vi "Raise WebMessage Received Event.vi"(4 "Event in":refnum<user-event>, 5 "Event Data":cluster{"sender":refnum<k24>, "e":refnum<k24>}, 6 "Control Ref":refnum<k24>, 7 "Event Common Data":T1) -> ()   [LabVIEW 2020, in "WebView.lvclass"]
uses:
  WebView.lvclass
  <vilib>/sklein/WebView2/Libs/Microsoft.Web.WebView2.Core.dll
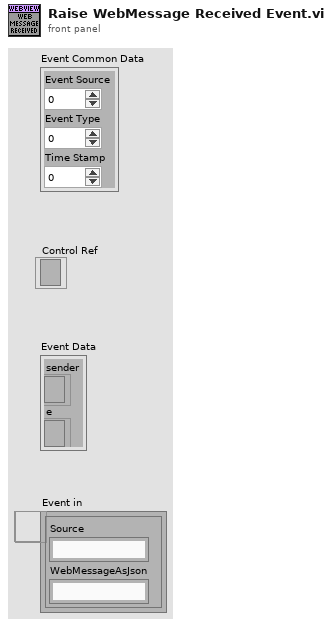
[diagram p1: front panel]
types:
  T1 = cluster{"Event Source":i32, "Event Type":u32, "Time Stamp":u32}
  T2 = cluster{"Source":string, "WebMessageAsJson":string}
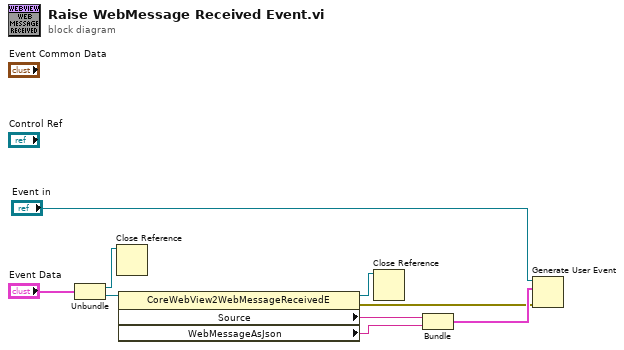
[diagram p0: block diagram]
diagram:
  n1 = Unbundle("Event Data") -> ("sender"=w3:refnum<k24>, "e"=w8:refnum<k24>)
  n2 = Close Reference(reference=w3) -> ()  [unwired: 1 in, 1 out]
  n3 = property class="CoreWebView2WebMessageReceivedE"(reference=w8) -> (reference out=w2:refnum<k24>, error out=w4:errorcluster, "Source"=w7:string, "WebMessageAsJson"=w6:string)  [unwired: 1 in]
  n4 = Close Reference(reference=w2) -> ()  [unwired: 1 in, 1 out]
  n5 = Bundle("Source"=w7, "WebMessageAsJson"=w6) -> (w5:T2)  [unwired: 1 in]
  n6 = Generate User Event(user event="Event in", event data cluster=w5, error in=w4) -> ()  [unwired: 1 in, 2 out]
